vi "SliceClass.vi"(8 "error in (no error)":errorcluster, 10 "Slicing":T3, 11 "SerializedClassHeader (child,parent)":T1[](array[typedef])) -> (0 "error IO":errorcluster, 2 "NumLevelsSliced":u16, 3 "from object (default value)":refnum<class>)   [LabVIEW 2019, in "BlueSerialization.lvlib" / "BlueSerializer.lvclass"]
uses:
  BlueSerializer.lvclass
  DeserializeSlicingOptions.ctl
  ClassHeader.ctl
  <vilib>/Utility/EditLVLibs/LibVersion.ctl
  <vilib>/Utility/error.llb/Error Cluster From Error Code.vi
  <vilib>/ErrorRing/Error Ring.xnode
  <vilib>/Utility/EditLVLibs/Edit LVLibs.lvlib
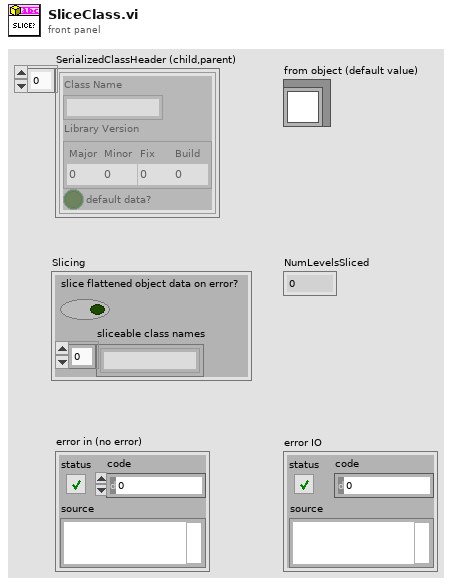
[diagram p1: front panel]
types:
  T1 = typedef "BlueSerialization.lvlib/BlueSerializer.lvclass/ClassHeader.ctl" = cluster{"Class Name":string, "Library Version":T2, "default data?":bool}
  T2 = typedef "Edit LVLibs.lvlib/LibVersion.ctl" = cluster{"Major":u16, "Minor":u16, "Fix":u16, "Build":u16}
  T3 = typedef "BlueSerialization.lvlib/BlueSerializer.lvclass/DeserializeSlicingOptions.ctl" = cluster{"slice flattened object data on error?":bool, "sliceable class names":string[]}
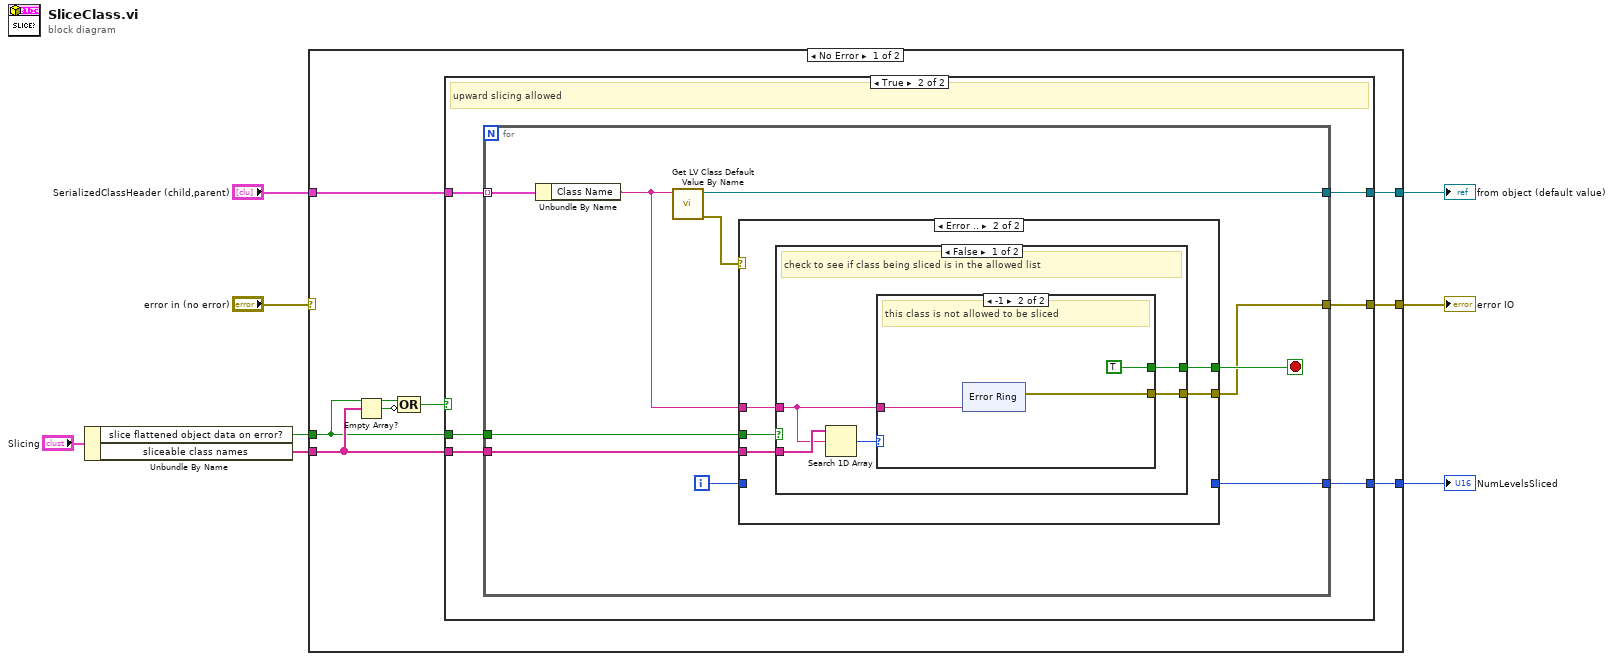
[diagram p0: block diagram]
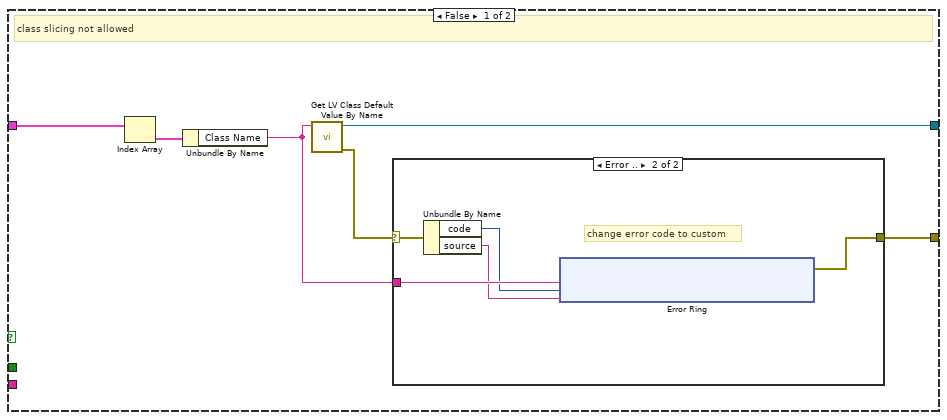
[diagram p2: hidden frame]
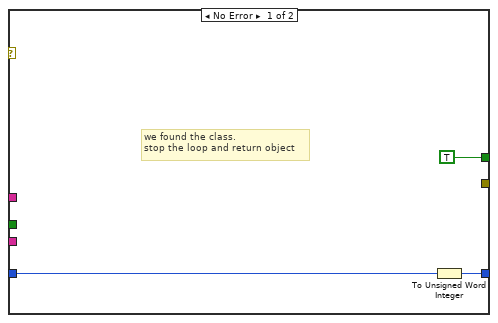
[diagram p4: hidden frame]
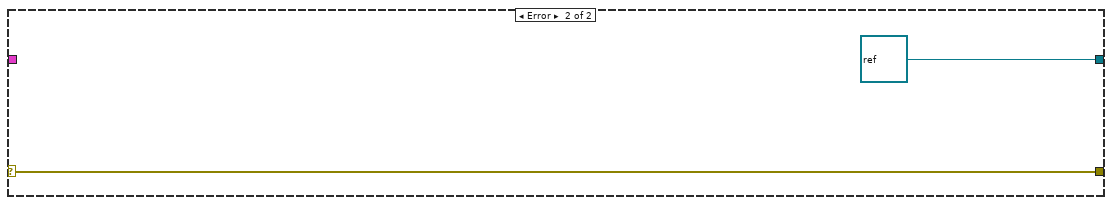
[diagram p7: hidden frame]
diagram:
  n1 = Unbundle By Name("Slicing") -> ("slice flattened object data on error?"=w7:bool, "sliceable class names"=w6:string[])
  n2 = case shown="No Error" "error in (no error)" {
    selector: "error in (no error)" -> [_ w78]
    tunnel: "SerializedClassHeader (child,parent)" -> [w16 _]
    tunnel: [w15 refnum<class> refnum ("object")] -> w4
    tunnel: [w14 w78] -> w3
    tunnel: w7 -> [w10 _]
    tunnel: w6 -> [w13 _]
    tunnel: [w9 _] -> w1
    frame No Error {
      n3 = Empty Array?(array=w13) -> (empty?=w11:bool)
      n4 = Compound Arithmetic op=OR(w10, invert w11) -> (w12:bool)
      n5 = case shown="True" w12 {
        tunnel: w16 -> [w19 w43]
        tunnel: [w22 w42] -> w15
        tunnel: [w21 w41] -> w14
        tunnel: w13 -> [_ w40]
        tunnel: w10 -> [_ w39]
        tunnel: [_ w38] -> w9
        frame False {
          # "class slicing not allowed"
          n6 = Index Array(array=w19) -> (element=w18:T1)  [unwired: 1 in]
          n7 = Unbundle By Name(w18) -> ("Class Name"=w17:string)
          n8 = call <vilib>:"Get LV Class Default Value By Name.vi"("class name"=w17) -> ("error out"=w20:errorcluster, "object"=w22:refnum<class>)  [unwired: 9 in]
          n9 = case shown="Error .." w20 {
            selector: w20 -> [w23 w26]
            tunnel: w17 -> [_ w28]
            tunnel: [w23 w27] -> w21
            frame No Error {
            }
            frame Error {
              # "change error code to custom"
              n10 = Unbundle By Name(w26) -> ("code"=w25:i32, "source"=w24:string)
              n11 = xnode "Error Ring"("parameter 0"=w28, "parameter 1"=w25, "parameter 2"=w24) -> ("error out"=w27:errorcluster)
            }
          }
        }
        frame True {
          # "upward slicing allowed"
          n12 = for {
            tunnel: w43 -> [w46] mode=indexing
            tunnel: [w52] -> w42
            tunnel: [w51] -> w41
            tunnel: w40 -> [w50]
            tunnel: w39 -> [w49]
            tunnel: [w47] -> w38
            i -> [w44]
            stop <- w53 stop-if-true
            n13 = Unbundle By Name(w46) -> ("Class Name"=w45:string)
            n14 = call <vilib>:"Get LV Class Default Value By Name.vi"("class name"=w45) -> ("error out"=w48:errorcluster, "object"=w52:refnum<class>)  [unwired: 9 in]
            n15 = case shown="Error .." w48 {
              tunnel: [TRUE w60] -> w53
              tunnel: w50 -> [_ w59]
              tunnel: w49 -> [_ w61]
              tunnel: w45 -> [_ w58]
              tunnel: [_ w57] -> w51
              tunnel: [w54 _] -> w47
              tunnel: w44 -> [w55 _]
              frame No Error {
                # "we found the class.\nstop the loop and return object"
                n16 = To Unsigned Word Integer(number=w55) -> (unsigned 16bit integer=w54:u16)
              }
              frame Error {
                n17 = case shown="False" w61 {
                  tunnel: [w64 _] -> w60
                  tunnel: w59 -> [w66 _]
                  tunnel: w58 -> [w63 _]
                  tunnel: [w62 _] -> w57
                  frame False {
                    # "check to see if class being sliced is in the allowed list"
                    n18 = Search 1D Array(1D array=w66, element=w63) -> (index of element=w65:i32)  [unwired: 1 in]
                    n19 = case shown="-1" w65 {
                      tunnel: [_ TRUE] -> w64
                      tunnel: w63 -> [_ w68]
                      tunnel: [_ w67] -> w62
                      frame Default {
                        # "keep trying"
                        # "slice-allowed class"
                      }
                      frame -1 {
                        # "this class is not allowed to be sliced"
                        n20 = xnode "Error Ring"("parameter 0"=w68) -> ("error out"=w67:errorcluster)
                      }
                    }
                  }
                  frame True {
                    # "Allow slicing of any class"
                  }
                }
              }
            }
          }
        }
      }
    }
    frame Error {
    }
  }
  "from object (default value)" <- w4
  "error IO" <- w3
  "NumLevelsSliced" <- w1
